vi "Measure.vi"(8 "error in":errorcluster, 11 "DIG_IO in":refnum<class "DIG_IO.lvclass">) -> (0 "error out":errorcluster, 3 "DIG_IO out":refnum<class "DIG_IO.lvclass">)   [LabVIEW 2019, in "DIG_IO.lvlib" / "DIG_IO.lvclass"]
uses:
  Library/DIG_IO.lvclass
  Library/DIG_IO.lvclass/DIG_IO.ctl
  builds/Instruments/Instruments.lvlibp/Library/Instruments.lvclass
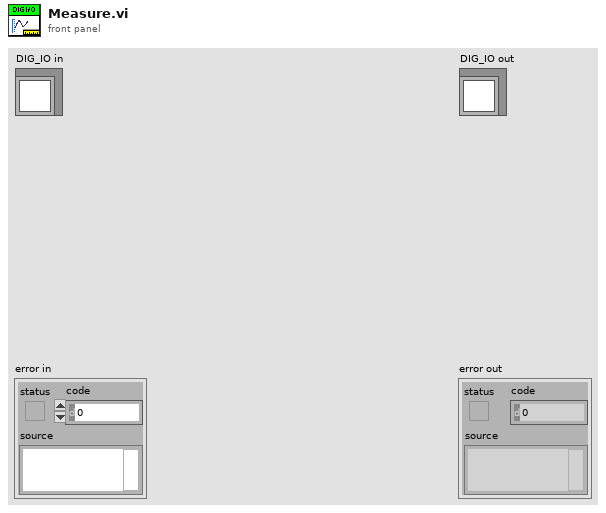
[diagram p1: front panel]
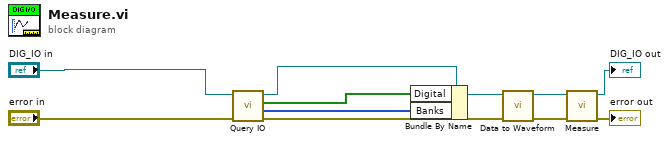
[diagram p0: block diagram]
diagram:
  n1 = call-dynamic "Query IO.vi"("error in"="error in", "DIG_IO in"="DIG_IO in") -> ("error out"=w7:errorcluster, "Port Array"=w1:u8[], "Boolean Array"=w2:bool[], "DIG_IO out"=w6:refnum<class "DIG_IO.lvclass">)  [unwired: 6 in]
  n2 = Bundle By Name(cluster=w6, "Digital"=w2, "Banks"=w1) -> (w3:refnum<class "DIG_IO.lvclass">)
  n3 = call "Data to Waveform.vi"("error in"=w7, "DIG_IO in"=w3) -> ("error out"=w4:errorcluster, "DIG_IO out"=w5:refnum<class "DIG_IO.lvclass">)  [unwired: 8 in]
  n4 = call-parent "Measure.vi"("error in"=w4, "Instruments in"=w5) -> ("error out"=→"error out":errorcluster, "Instruments out"=→"DIG_IO out":refnum<class "DIG_IO.lvclass">)  [unwired: 8 in]
